vi "color_scheme.vi"() -> ()   [LabVIEW 2015, in "blog-lv-interface-prototype.lvlib"]
uses:
  blog-lv-interface-prototype.lvlib
panel:
  in  "pipe 3":bool=TRUE caption="pipe"
  in  "pipe 2":bool=TRUE caption="pipe"
  in  "pipe":bool=TRUE
  # "Build Interface"
  # "Sample"
  # "Sample"
  # "SAMPLE"
  # "SAMPLE"
  # "sample"
  # "sample"
  # "Build Interface"
  # "Sample"
  # "Sample"
  # "SAMPLE"
  # "SAMPLE"
  # "sample"
  # "sample"
  # "Build Interface"
  # "Sample"
  # "Sample"
  # "SAMPLE"
  # "SAMPLE"
  # "sample"
  # "sample"
  # "R: 15\nG: 93\nB: 44"
  # "R: 128\nG: 40\nB: 21"
  # "R: 218\nG: 218\nB: 218"
  # "R: 170\nG: 89\nB: 57"
  # "R: 39\nG: 117\nB: 83"
  # "R: 37\nG: 37\nB: 37"
  # "R: 45\nG: 70\nB: 113"
  # "R: 170\nG: 130\nB: 57"
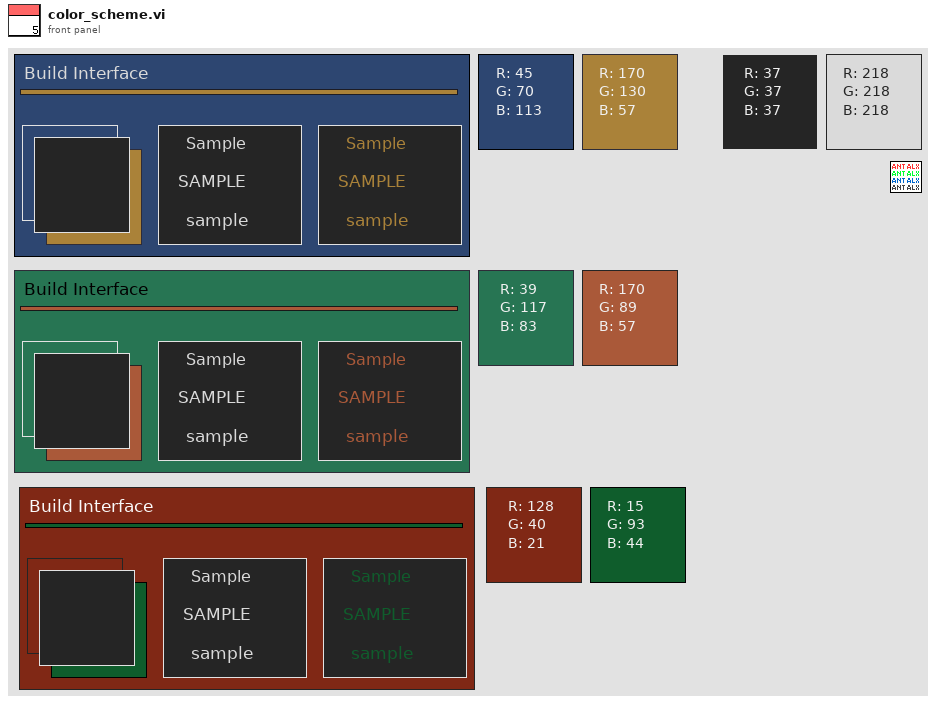
[diagram p1: front panel]
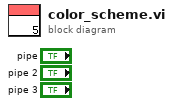
[diagram p0: block diagram]
diagram:
